vi "Register Load Pressed.vi"(8 "error in (no error)":errorcluster, 11 "UI Controller in":refnum<class "UI Controller.lvclass">) -> (0 "error out":errorcluster, 3 "UI Controller out":refnum<class "UI Controller.lvclass">)   [LabVIEW 2020, in "UI Controller.lvlib" / "UI Controller.lvclass"]
uses:
  UI Controller.lvclass
  C:/Program Files/National Instruments/LabVIEW 2020/vi.lib/ActorFrameworkMVC/Abstract Controller/Abstract Controller/Abstract Controller.lvclass
  C:/Program Files/National Instruments/LabVIEW 2020/vi.lib/ActorFramework/Actor/Actor.lvclass
  Views/Side Menu View/Side Menu View Messages/Register Load Pressed Msg/Register Load Pressed Msg.lvclass
  C:/Program Files/National Instruments/LabVIEW 2020/vi.lib/ActorFramework/Message/Message.lvclass
  Models/Yaml Model/Yaml Model Messages/Concrete Load Pressed Msg/Concrete Load Pressed Msg.lvclass
  C:/Program Files/National Instruments/LabVIEW 2020/vi.lib/ActorFrameworkObserver/Data Message/Data Message.lvclass
  <vilib>/ActorFramework/Message Enqueuer/Message Enqueuer.lvclass/Message Enqueuer.ctl
  UI Controller Messages/Concrete Load Pressed Msg/Concrete Load Pressed Msg.lvclass
  <vilib>/ActorFramework/Actor/Actor.lvclass/Actor.ctl
  <vilib>/ActorFramework/Message Enqueuer/Init from Existing Queue.vi
  <vilib>/ActorFramework/Message Priority Queue/Priority Enqueue.vi
  <vilib>/ActorFramework/Message Enqueuer/Message Enqueuer.lvclass
  <vilib>/ActorFrameworkMVC/Abstract Controller/Abstract Controller/Abstract Controller.lvclass
  <vilib>/ActorFramework/Actor/Actor.lvclass
panel:
  # "NOTICE -- YOU MUST LEAVE THIS NOTICE IN PLACE.\n\nCopyright (c) 2017, LIANG LIU Shawn.Liu.cn@gmail.com\nAll rights reserved.\n\nRedistribution and use in source and binary forms, with or without modification, are permitted provided that the following conditions are met:\n-Redistributions of source code must retain the above copyright notice, this list of conditions and the following disclaimer.\n-Redistributions in binary form must reproduce the above copyright notice, this list of conditions and the following disclaimer in the documentation and/or other materials provided with the distribution.\n-Neither the name of the eLp nor the names of its contributors may be used to endorse or promote products derived from this software without specific prior written permission.\n\nTHIS SOFTWARE IS PROVIDED BY THE COPYRIGHT HOLDERS AND CONTRIBUTORS \"AS IS\" AND ANY EXPRESS OR IMPLIED WARRANTIES, INCLUDING, BUT NOT LIMITED TO, THE IMPLIED WARRANTIES OF MERCHANTABILITY AND FITNESS FOR A PARTICULAR PURPOSE ARE DISCLAIMED. IN NO EVENT SHALL THE COPYRIGHT HOLDER OR CONTRIBUTORS BE LIABLE FOR ANY DIRECT, INDIRECT, INCIDENTAL, SPECIAL, EXEMPLARY, OR CONSEQUENTIAL DAMAGES (INCLUDING, BUT NOT LIMITED TO, PROCUREMENT OF SUBSTITUTE GOODS OR SERVICES; LOSS OF USE, DATA, OR PROFITS; OR BUSINESS INTERRUPTION) HOWEVER CAUSED AND ON ANY THEORY OF LIABILITY, WHETHER IN CONTRACT, STRICT LIABILITY, OR TORT (INCLUDING NEGLIGENCE OR OTHERWISE) ARISING IN ANY WAY OUT OF THE USE OF THIS SOFTWARE, EVEN IF ADVISED OF THE POSSIBILITY OF SUCH DAMAGE."
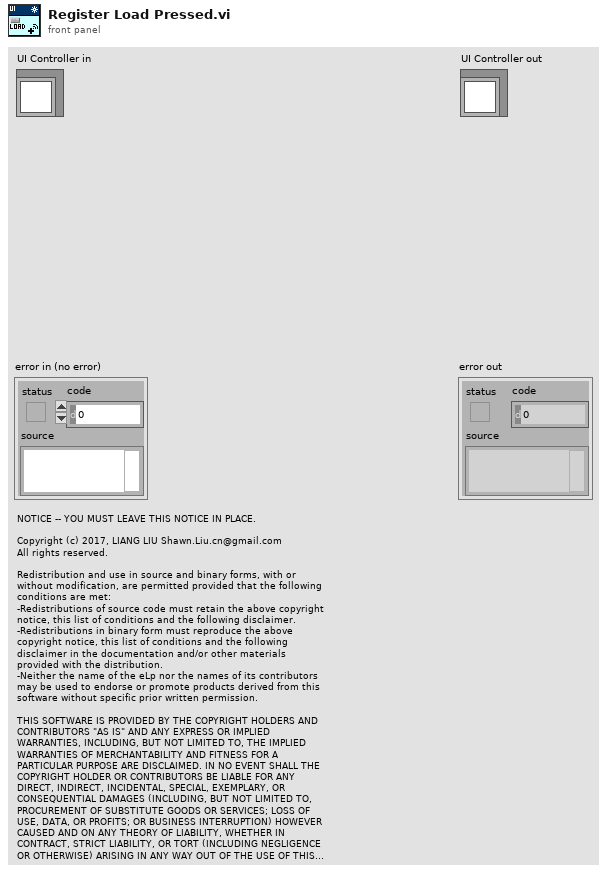
[diagram p1: front panel]
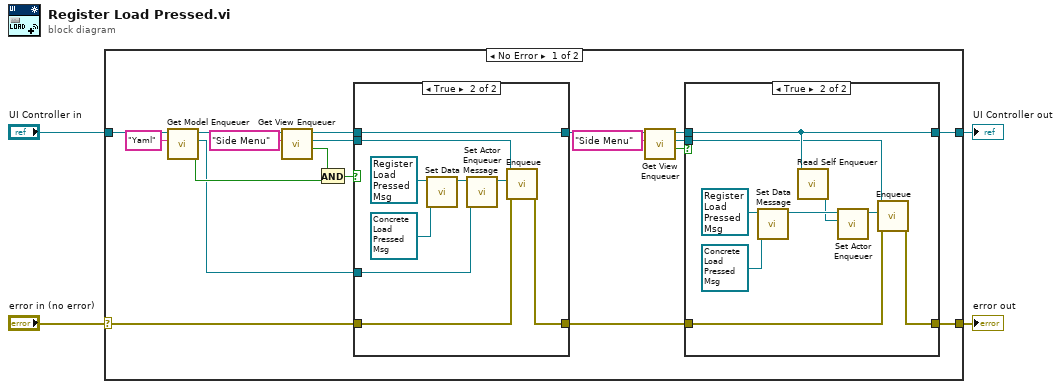
[diagram p0: block diagram]
diagram:
  n1 = case shown="No Error" "error in (no error)" {
    selector: "error in (no error)" -> [w22 w47]
    tunnel: "UI Controller in" -> [w23 w46]
    tunnel: [w7 w46] -> w2
    tunnel: [w6 w47] -> w1
    frame No Error {
      n2 = call <vilib>:"Get Model Enqueuer.vi"("Model Name"="Yaml", "Abstract Controller in"=w23) -> ("Found?"=w14:bool, "Model Enqueuer"=w13:refnum<class "Message Enqueuer.lvclass">, "Abstract Controller out"=w18:refnum<class "UI Controller.lvclass">)  [unwired: 6 in, 1 out]
      n3 = call <vilib>:"Get View Enqueuer.vi"("View Name"="Side Menu", "Abstract Controller in"=w18) -> ("Found?"=w15:bool, "View Enqueuer"=w20:refnum<class "Message Enqueuer.lvclass">, "Abstract Controller out"=w19:refnum<class "UI Controller.lvclass">)  [unwired: 6 in, 1 out]
      n4 = And(x=w15, y=w14) -> (x .and. y?=w16:bool)
      n5 = case shown="True" w16 {
        tunnel: w20 -> [_ w41]
        tunnel: w19 -> [w36 w42]
        tunnel: [w36 w42] -> w8
        tunnel: w22 -> [w35 w39]
        tunnel: [w35 w38] -> w5
        tunnel: w13 -> [_ w37]
        frame False {
        }
        frame True {
          n6 = call-dynamic "Set Data Message.vi"("Data Message"=refnum<class "Concrete Load Pressed Msg.lvclass"> refnum ("Yaml Model.lvlib:Concrete Load Pressed Msg.lvclass"), "Registration Message in"=refnum<class "Register Load Pressed Msg.lvclass"> refnum ("Side Menu View.lvlib:Register Load Pressed Msg.lvclass")) -> ("Registration Message out"=w44:refnum<class "Register Load Pressed Msg.lvclass">)  [unwired: 9 in]
          n7 = call-dynamic "Set Actor Enqueuer.vi"("Actor Enqueuer"=w37, "Registration Message in"=w44) -> ("Registration Message out"=w40:refnum<class "Register Load Pressed Msg.lvclass">)  [unwired: 9 in]
          n8 = call <vilib>:"Enqueue.vi"("error in (no error)"=w39, "Message"=w40, "Message Enqueuer in"=w41) -> ("error out"=w38:errorcluster)  [unwired: 7 in, 1 out]
        }
      }
      n9 = call <vilib>:"Get View Enqueuer.vi"("View Name"="Side Menu", "Abstract Controller in"=w8) -> ("Found?"=w11:bool, "View Enqueuer"=w10:refnum<class "Message Enqueuer.lvclass">, "Abstract Controller out"=w9:refnum<class "UI Controller.lvclass">)  [unwired: 6 in, 1 out]
      n10 = case shown="True" w11 {
        tunnel: w10 -> [_ w29]
        tunnel: w9 -> [w25 w30]
        tunnel: [w25 w30] -> w7
        tunnel: w5 -> [w24 w27]
        tunnel: [w24 w26] -> w6
        frame False {
        }
        frame True {
          n11 = call-dynamic "Set Data Message.vi"("Data Message"=refnum<class "Concrete Load Pressed Msg.lvclass"> refnum ("UI Controller.lvlib:Concrete Load Pressed Msg.lvclass"), "Registration Message in"=refnum<class "Register Load Pressed Msg.lvclass"> refnum ("Side Menu View.lvlib:Register Load Pressed Msg.lvclass")) -> ("Registration Message out"=w33:refnum<class "Register Load Pressed Msg.lvclass">)  [unwired: 9 in]
          n12 = call <vilib>:"Read Self Enqueuer.vi"("Actor"=w30) -> ("Self Enqueuer"=w31:refnum<class "Message Enqueuer.lvclass">)  [unwired: 10 in]
          n13 = call-dynamic "Set Actor Enqueuer.vi"("Actor Enqueuer"=w31, "Registration Message in"=w33) -> ("Registration Message out"=w28:refnum<class "Register Load Pressed Msg.lvclass">)  [unwired: 9 in]
          n14 = call <vilib>:"Enqueue.vi"("error in (no error)"=w27, "Message"=w28, "Message Enqueuer in"=w29) -> ("error out"=w26:errorcluster)  [unwired: 7 in, 1 out]
        }
      }
    }
    frame Error {
    }
  }
  "error out" <- w1
  "UI Controller out" <- w2
